vi "Leaderboard export.vi"(10 "current time":timestamp, 11 "path to PNG file":path) -> (0 "error out":errorcluster, 3 "path":path)   [LabVIEW 2020, in "Visualisation.lvclass"]
uses:
  Visualisation.lvclass
  Application/Globals.vi
  Data Manager/Data Manager.lvclass
  Application/Application.lvlib
panel:
  in  "Export":enum32{"Page 1", "Page 2"}(tab)
  out "B Lead":dbl format="+ %0.1f km"
  out "A Lead":dbl format="+ %0.1f km"
  out "A Total":dbl format="%0.1f km"
  out "B Total":dbl format="%0.1f km"
  out "Run":T1(array[cluster]) {"Distance 2" scale=0.0..96.2213}
  out "Ride":T2(array[cluster]) {"Distance 4" scale=0.0..76.5197}
  out "Leaderboard":T3(array[cluster]) {"Distance" scale=0.0..167.7288}
  out "Walk":T1(array[cluster]) {"Distance 2" scale=0.0..92.6965}
  out "Group Totals 1":dbl format="%0.1f km"
  out "Group Totals 2":dbl format="%0.1f km"
  out "Line 1":string
  out "Group Totals 3":dbl format="%0.1f km"
  out "Group Totals 4":dbl format="%0.1f km"
  out "Line 2":string
  out "Group Totals 5":dbl format="%0.1f km"
  out "Group Totals 6":dbl format="%0.1f km"
  out "Line 3":string
  out "Table Control":string[][](table)
  out "Daily Change A":dbl format="+ %0.1f km"
  out "Daily Change B":dbl format="+ %0.1f km"
  # "Total Distance Leaderboard"
  # "Head to Head"
  # "VS"
  # "VS"
  # "VS"
  # "Longest Single Activity"
  # "Daily Total Distance Change"
  # "VS"
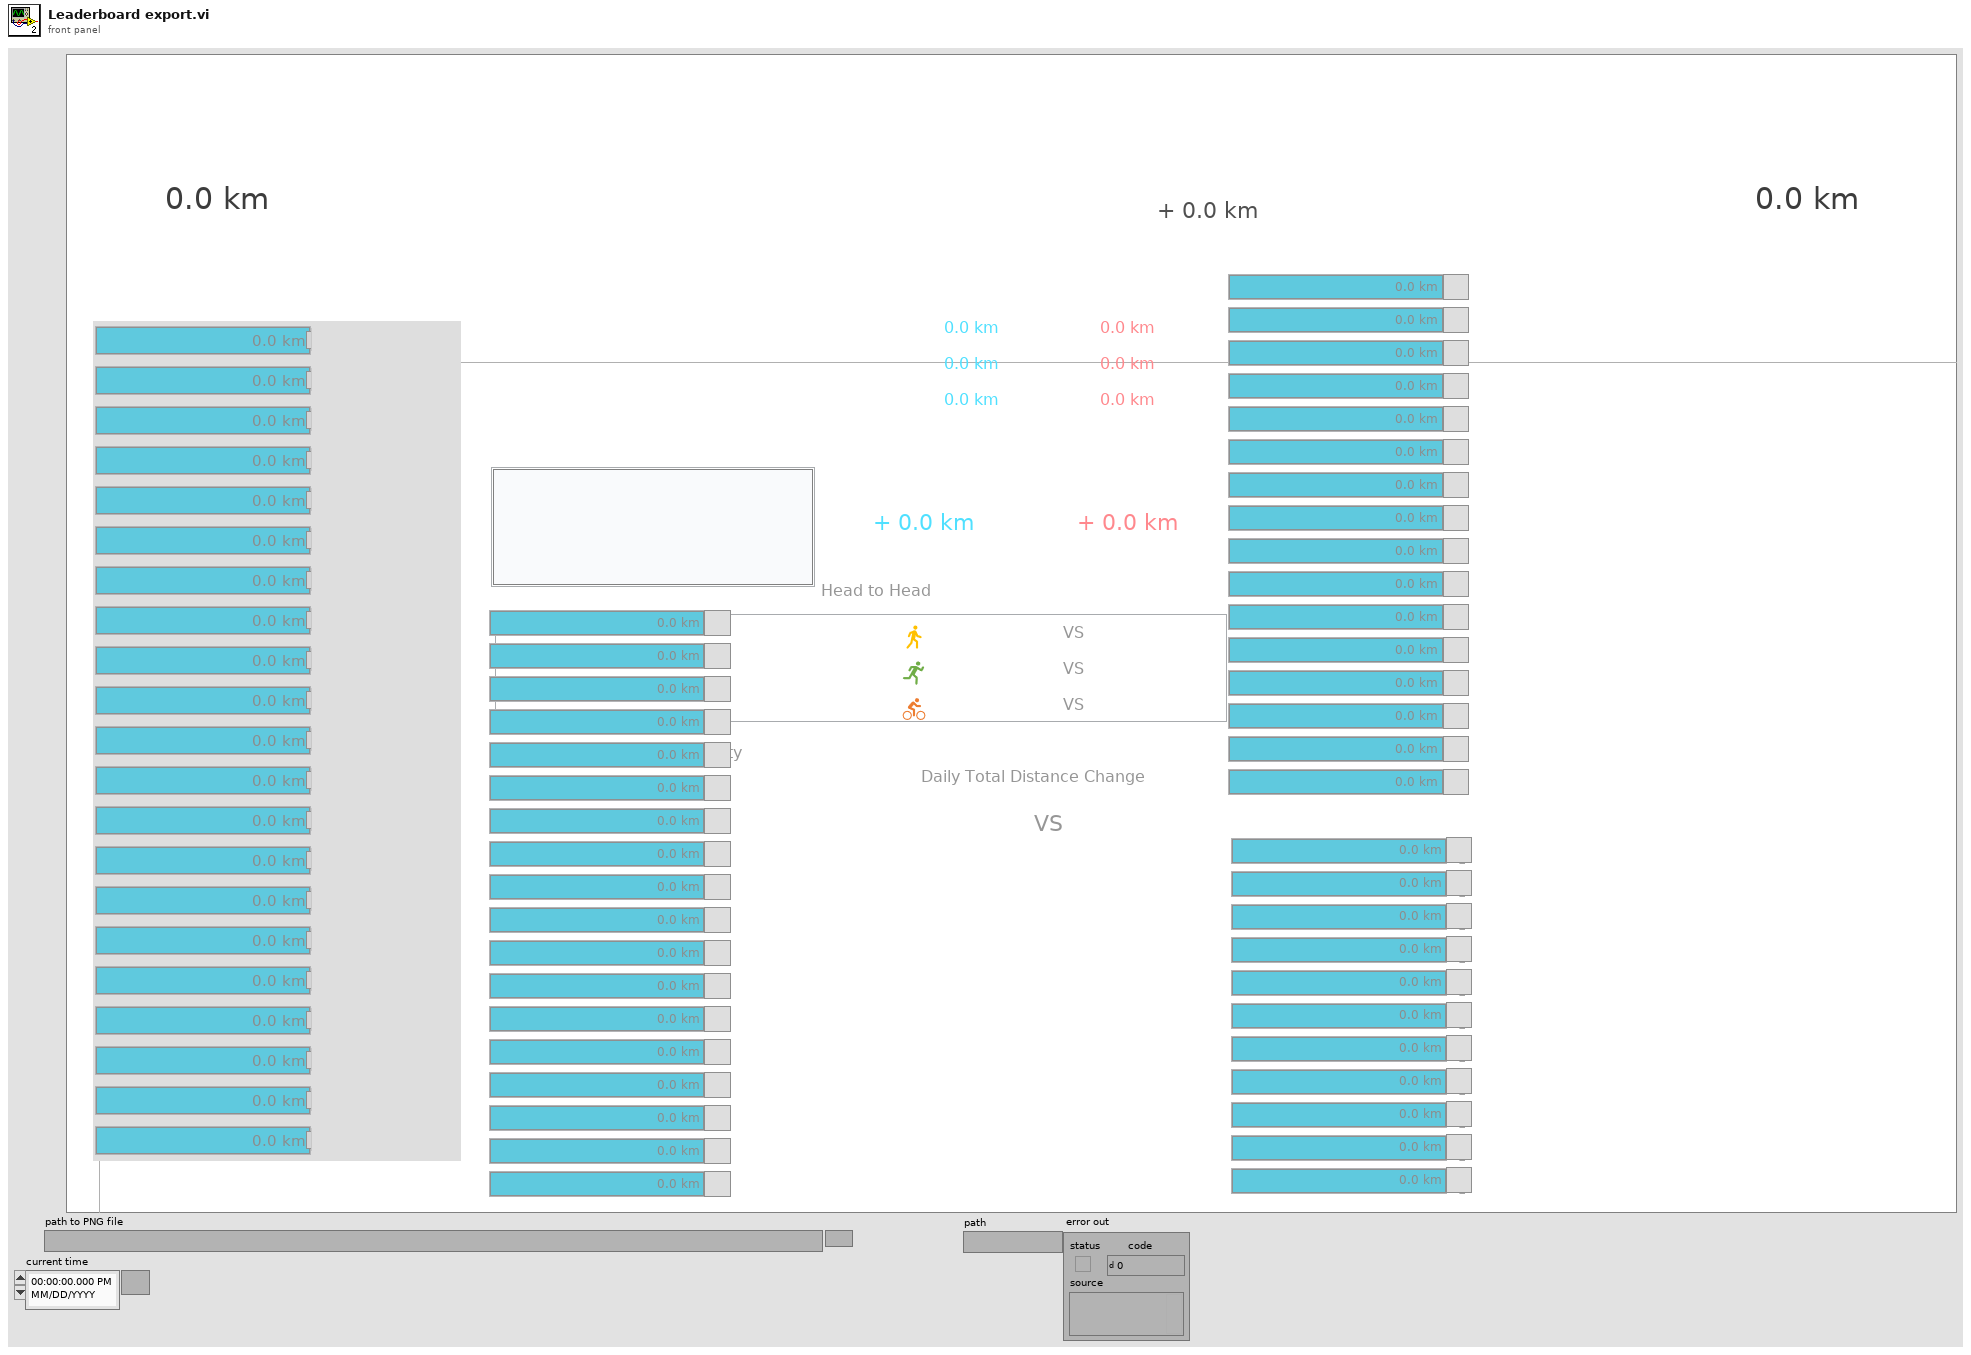
[diagram p1: front panel]
types:
  T1 = cluster{"Athlete":string, "Team":u32, "Distance 2":dbl}[]
  T2 = cluster{"Athlete":string, "Team":u32, "Distance 4":dbl}[]
  T3 = cluster{"Athlete":string, "Distance":dbl, "Team":u32}[]
  T4 = cluster{"Athlete":string, "Distance":dbl, "Team":u32}
  T5 = cluster{"Athlete":string, "Team":u32, "Distance 2":dbl}
  T6 = cluster{"Athlete":string, "Distance":dbl, "Team":u32, "Distance 2":cluster{"Numeric":dbl, "Numeric":dbl, "Numeric":dbl}}
  T7 = typedef "imagedata.ctl" = cluster{"image type":i32, "image depth":i32, "image":u8[], "mask":u8[], "colors":u32[], "Rectangle":cluster{"left":i16, "top":i16, "right":i16, "bottom":i16}}
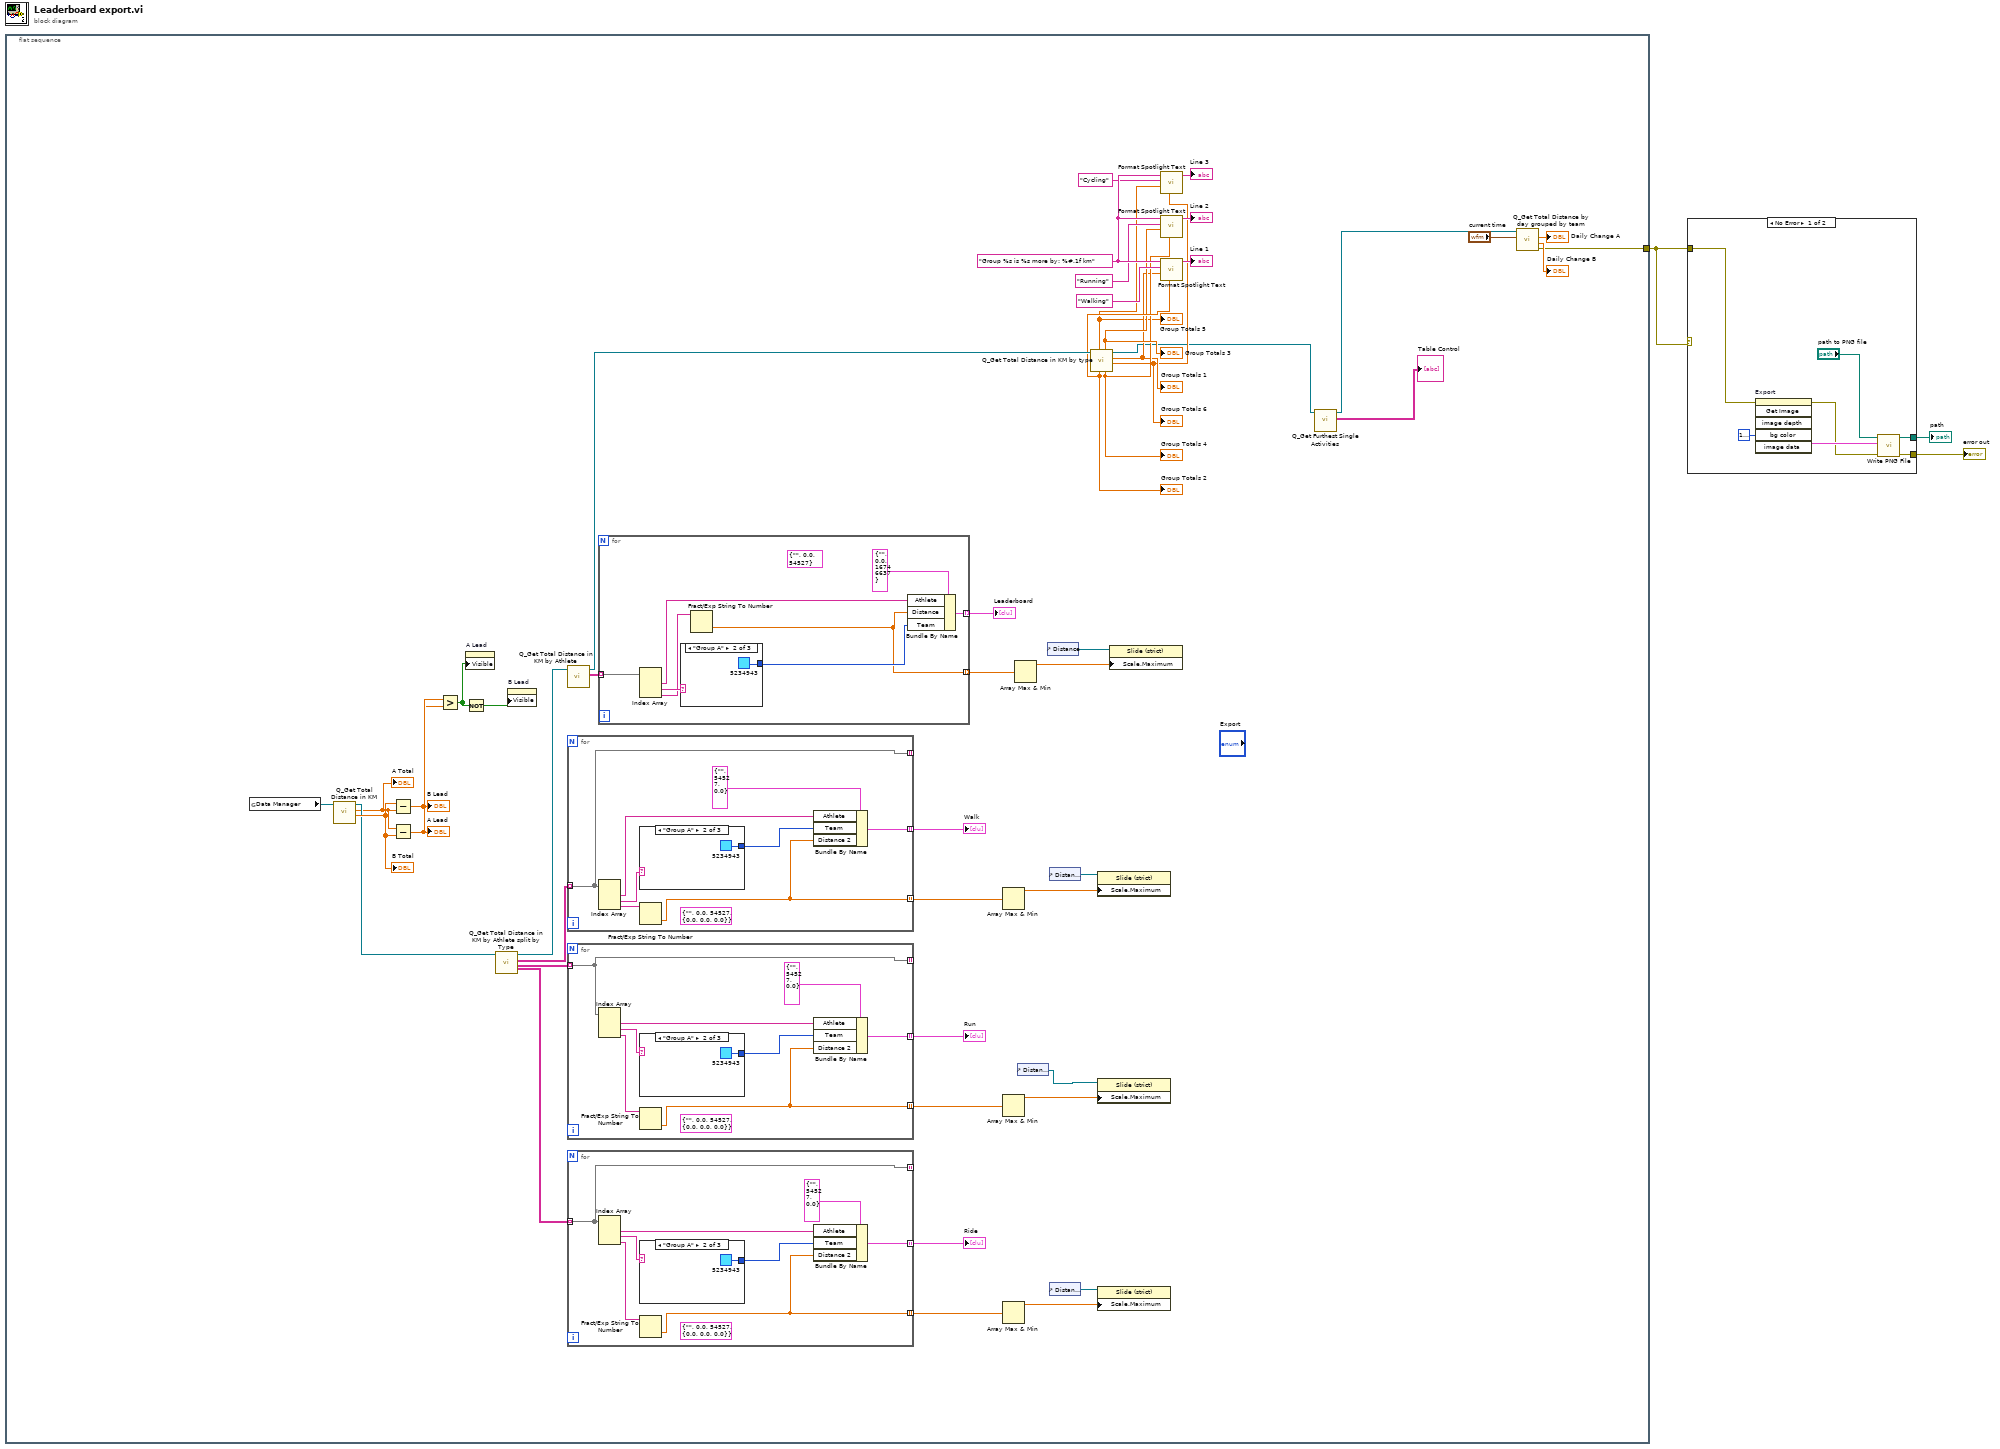
[diagram p0: block diagram]
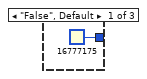
[diagram p3: hidden frame]
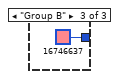
[diagram p4: hidden frame]
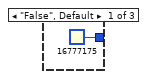
[diagram p5: hidden frame]
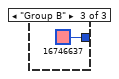
[diagram p6: hidden frame]
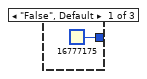
[diagram p7: hidden frame]
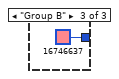
[diagram p8: hidden frame]
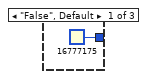
[diagram p9: hidden frame]
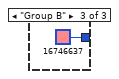
[diagram p10: hidden frame]
diagram:
  n1 = flat-sequence {
    tunnel: [w5] -> w1
    frame #0 {
      w27 = "Group %s is %s more by: %#.1f km"
      n2 = global read "Globals.vi" "Data Manager"() -> (w53:refnum<class "Data Manager.lvclass">)
      n3 = call-dynamic "Q_Get Total Distance in KM.vi"("Data Manager in"=w53) -> ("Group B"=w12:dbl, "Group A"=w10:dbl, "Data Manager out"=w11:refnum<class "Data Manager.lvclass">)  [unwired: 6 in, 2 out]
      "A Total" <- w10
      "B Total" <- w12
      n4 = Subtract(x=w12, y=w10) -> (x-y=w8:dbl)
      "B Lead" <- w8
      n5 = Subtract(x=w10, y=w12) -> (x-y=w9:dbl)
      "A Lead" <- w9
      n6 = Greater?(x=w9, y=w8) -> (0:w7:bool)
      n7 = Not(x=w7) -> (.not. x?=w6:bool)
      n8 = property on="A Lead" class="DigNum (strict)"("Visible"=w7) -> ()  [unwired: 2 in, 2 out]
      n9 = call-dynamic "Q_Get Total Distance in KM by Athlete split by Type.vi"("Data Manager in"=w11) -> ("Run"=w46:string[][], "Walk"=w50:string[][], "Data Manager out"=w39:refnum<class "Data Manager.lvclass">, "Ride"=w43:string[][])  [unwired: 6 in, 1 out]
      n10 = property on="B Lead" class="DigNum (strict)"("Visible"=w6) -> ()  [unwired: 2 in, 2 out]
      n11 = call-dynamic "Q_Get Total Distance in KM by Athlete.vi"("Data Manager in"=w39) -> ("Result Set"=w38:string[][], "Data Manager out"=w31:refnum<class "Data Manager.lvclass">)  [unwired: 8 in, 1 out]
      n12 = for {
        tunnel: [w89] -> _ mode=indexing
        tunnel: [w94] -> w33 mode=indexing
        tunnel: w50 -> [w89] mode=indexing
        tunnel: [w88] -> w47 mode=indexing
        (unwired) T6 {"Athlete"="", "Distance"=0.0, "Team"=54527, "Distance 2"={"Numeric"=0.0, "Numeric"=0.0, "Numeric"=0.0}} ("Leaderboard")
        n13 = Index Array(array=w89) -> (element #1=w90:string, element #2=w92:string, element #3=w91:string)  [unwired: 3 in]
        n14 = case shown="\"Group A\"" w92 {
          tunnel: [u32 16777175 ("Color Box") u32 5234943 ("Color Box") u32 16746637 ("Color Box")] -> w93
          frame "False", Default {
          }
          frame "Group A" {
          }
          frame "Group B" {
          }
        }
        n15 = Fract/Exp String To Number(string=w91) -> (number=w88:dbl)  [unwired: 3 in, 1 out]
        n16 = Bundle By Name(cluster=T5 {"Athlete"="", "Team"=54527, "Distance 2"=0.0} ("Leaderboard"), "Athlete"=w90, "Team"=w93, "Distance 2"=w88) -> (w94:T5)
      }
      "Walk" <- w33
      n17 = for {
        tunnel: w46 -> [w78] mode=indexing
        tunnel: [w83] -> w44 mode=indexing
        tunnel: [w78] -> _ mode=indexing
        tunnel: [w77] -> w45 mode=indexing
        (unwired) T6 {"Athlete"="", "Distance"=0.0, "Team"=54527, "Distance 2"={"Numeric"=0.0, "Numeric"=0.0, "Numeric"=0.0}} ("Leaderboard")
        n18 = Index Array(array=w78) -> (element #1=w79:string, element #2=w81:string, element #3=w80:string)  [unwired: 3 in]
        n19 = case shown="\"Group A\"" w81 {
          tunnel: [u32 16777175 ("Color Box") u32 5234943 ("Color Box") u32 16746637 ("Color Box")] -> w82
          frame "False", Default {
          }
          frame "Group A" {
          }
          frame "Group B" {
          }
        }
        n20 = Fract/Exp String To Number(string=w80) -> (number=w77:dbl)  [unwired: 3 in, 1 out]
        n21 = Bundle By Name(cluster=T5 {"Athlete"="", "Team"=54527, "Distance 2"=0.0} ("Leaderboard"), "Athlete"=w79, "Team"=w82, "Distance 2"=w77) -> (w83:T5)
      }
      "Run" <- w44
      n22 = for {
        tunnel: w43 -> [w67] mode=indexing
        tunnel: [w72] -> w41 mode=indexing
        tunnel: [w67] -> _ mode=indexing
        tunnel: [w66] -> w42 mode=indexing
        (unwired) T6 {"Athlete"="", "Distance"=0.0, "Team"=54527, "Distance 2"={"Numeric"=0.0, "Numeric"=0.0, "Numeric"=0.0}} ("Leaderboard")
        n23 = Index Array(array=w67) -> (element #1=w68:string, element #2=w70:string, element #3=w69:string)  [unwired: 3 in]
        n24 = case shown="\"Group A\"" w70 {
          tunnel: [u32 16777175 ("Color Box") u32 5234943 ("Color Box") u32 16746637 ("Color Box")] -> w71
          frame "False", Default {
          }
          frame "Group A" {
          }
          frame "Group B" {
          }
        }
        n25 = Fract/Exp String To Number(string=w69) -> (number=w66:dbl)  [unwired: 3 in, 1 out]
        n26 = Bundle By Name(cluster=T5 {"Athlete"="", "Team"=54527, "Distance 2"=0.0} ("Leaderboard"), "Athlete"=w68, "Team"=w71, "Distance 2"=w66) -> (w72:T5)
      }
      "Ride" <- w41
      n27 = for {
        tunnel: w38 -> [w60] mode=indexing
        tunnel: [w61] -> w37 mode=indexing
        tunnel: [w54] -> w35 mode=indexing
        (unwired) T4 {"Athlete"="", "Distance"=0.0, "Team"=54527} ("Leaderboard")
        n28 = Index Array(array=w60) -> (element #1=w56:string, element #2=w58:string, element #3=w57:string)  [unwired: 3 in]
        n29 = case shown="\"Group A\"" w58 {
          tunnel: [u32 16777175 ("Color Box") u32 5234943 ("Color Box") u32 16746637 ("Color Box")] -> w59
          frame "False", Default {
          }
          frame "Group A" {
          }
          frame "Group B" {
          }
        }
        n30 = Fract/Exp String To Number(string=w57) -> (number=w54:dbl)  [unwired: 3 in, 1 out]
        n31 = Bundle By Name(cluster=T4 {"Athlete"="", "Distance"=0.0, "Team"=16746637} ("Leaderboard"), "Athlete"=w56, "Distance"=w54, "Team"=w59) -> (w61:T4)
      }
      "Leaderboard" <- w37
      n32 = Array Max & Min(array=w47) -> (max value=w48:dbl)  [unwired: 3 out]
      n33 = Array Max & Min(array=w45) -> (max value=w52:dbl)  [unwired: 3 out]
      n34 = Array Max & Min(array=w42) -> (max value=w51:dbl)  [unwired: 3 out]
      n35 = Array Max & Min(array=w35) -> (max value=w36:dbl)  [unwired: 3 out]
      n36 = control-ref of="Distance 2"() -> (w32:refnum<vi>)
      n37 = control-ref of="Distance"() -> (w34:refnum<vi>)
      n38 = control-ref of="Distance 2"() -> (w49:refnum<vi>)
      n39 = control-ref of="Distance 4"() -> (w40:refnum<vi>)
      n40 = call-dynamic "Q_Get Total Distance in KM by type.vi"("Data Manager in"=w31) -> ("B Ride"=w18:dbl, "A Walk"=w20:dbl, "Data Manager out"=w17:refnum<class "Data Manager.lvclass">, "Run"=w21:dbl, "A Run"=w22:dbl, "Walk"=w30:dbl, "A Ride"=w19:dbl)  [unwired: 3 in, 1 out]
      "Group Totals 1" <- w20
      "Group Totals 2" <- w30
      "Group Totals 3" <- w22
      "Group Totals 4" <- w21
      "Group Totals 5" <- w19
      "Group Totals 6" <- w18
      n41 = property on="Property Node" class="Slide (strict)"(reference=w49, "Scale.Maximum"=w48) -> ()  [unwired: 1 in, 2 out]
      n42 = property on="Property Node" class="Slide (strict)"(reference=w32, "Scale.Maximum"=w52) -> ()  [unwired: 1 in, 2 out]
      n43 = property on="Property Node" class="Slide (strict)"(reference=w40, "Scale.Maximum"=w51) -> ()  [unwired: 1 in, 2 out]
      n44 = property on="Property Node" class="Slide (strict)"(reference=w34, "Scale.Maximum"=w36) -> ()  [unwired: 1 in, 2 out]
      n45 = call "Format Spotlight Text.vi"("Walk"=w18, "A Walk"=w19, "String"="Cycling", "String 2"=w27) -> ("String 3"=→"Line 3":string)  [unwired: 7 in]
      n46 = call "Format Spotlight Text.vi"("Walk"=w21, "A Walk"=w22, "String"="Running", "String 2"=w27) -> ("String 3"=→"Line 2":string)  [unwired: 7 in]
      n47 = call "Format Spotlight Text.vi"("Walk"=w30, "A Walk"=w20, "String"="Walking", "String 2"=w27) -> ("String 3"=→"Line 1":string)  [unwired: 7 in]
      n48 = call-dynamic "Q_Get Furthest Single Activities.vi"("Data Manager in"=w17) -> ("Result Set"=→"Table Control":string[][], "Data Manager out"=w15:refnum<class "Data Manager.lvclass">)  [unwired: 8 in, 1 out]
      n49 = call-dynamic "Q_Get Total Distance by day grouped by team.vi"("current time"="current time", "Data Manager in"=w15) -> ("error out"=w5:errorcluster, "Group B Daily"=→"Daily Change B":dbl, "Group A Daily"=→"Daily Change A":dbl)  [unwired: 6 in, 1 out]
    }
  }
  n50 = case shown="No Error" w1 {
    tunnel: w1 -> [w102 _]
    tunnel: [w100 _] -> w3
    tunnel: [w99 _] -> w2
    frame No Error {
      n51 = invoke on="Export" class="TabCtl (strict)" method="Get Image"(error in=w102, "bg color"=u32 16777216 ("Background Color")) -> (error out=w98:errorcluster, "image data"=w103:T7)  [unwired: 4 in, 4 out]
      n52 = call <vilib>:"Write PNG File.vi"("error in (no error)"=w98, "image data"=w103, "path to PNG file"="path to PNG file") -> ("error out"=w99:errorcluster, "path"=w100:path)  [unwired: 7 in]
    }
    frame Error {
    }
  }
  "path" <- w3
  "error out" <- w2
